vi "Error Enqueue.vi"(6 "Priority?":bool, 8 "error in":errorcluster, 11 "Error Message in":refnum<class "Error.lvclass">) -> (0 "error out":errorcluster, 3 "Error Message out":refnum<class "Error.lvclass">)   [LabVIEW 2017, in "TSC Error.lvlib"]
doc: "Send an error message.\n\nInputs:\n-Error Message in [obj] - the dynamic dispatch input class that will be queued to the Error Loop\n-error in\n\nOutputs:\n-Error Message out [obj] - the dynamic dispatch class that was queued to the Error Loop\n-error out\n________________________________________________________________________________\n<b>Code Developed By:</b>\nDaniel Coons\nTechnology Service Corporation\n1983 S Liberty Drive\nBloomington, IN 47403\nPhone: 812 558-7100\ndaniel.coons@tsc.com\nwww.tsc.com\n\n<b>Date Created:</b> 11 AUG 2014\n<b>Date Updated:</b>"
uses:
  TSC Error.lvlib
  _Messages/Error/Error.lvclass
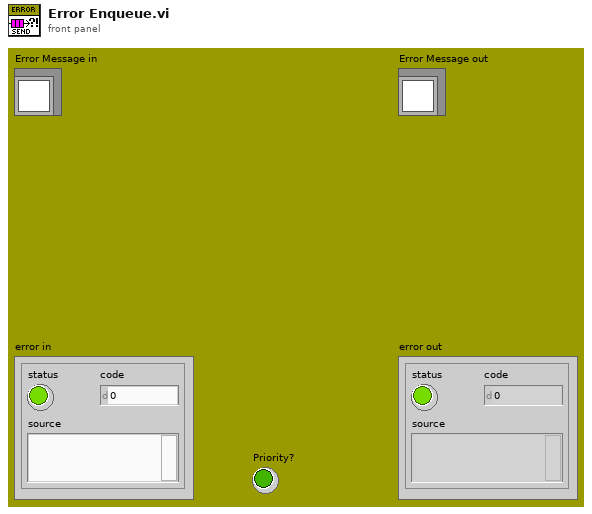
[diagram p1: front panel]
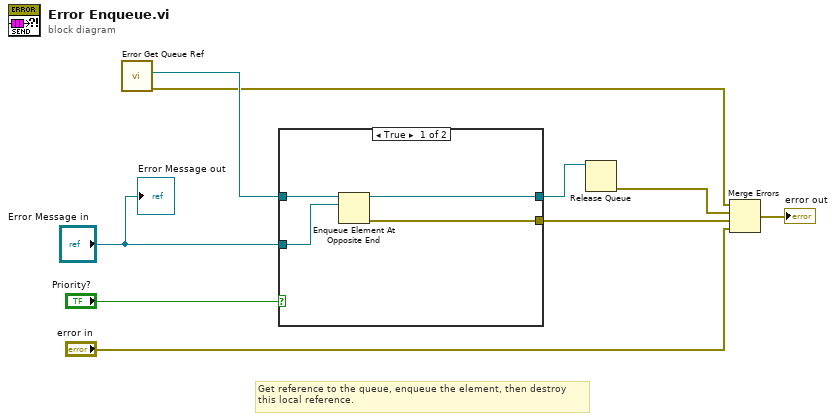
[diagram p0: block diagram]
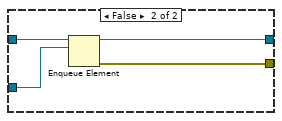
[diagram p2: hidden frame]
diagram:
  # "Get reference to the queue, enqueue the element, then destroy\nthis local reference."
  n1 = call "Error Get Queue Ref.vi"() -> ("error out"=w5:errorcluster, "Error Queue out"=w7:refnum<queue>)  [unwired: 9 in, 1 out]
  n2 = case shown="True" "Priority?" {
    tunnel: "Error Message in" -> [w13 w17]
    tunnel: [w12 w16] -> w4
    tunnel: [w11 w15] -> w8
    tunnel: w7 -> [w10 w14]
    frame True {
      n3 = Enqueue Element At Opposite End(queue=w10, element=w13) -> (queue out=w11:refnum<queue>, error out=w12:errorcluster)  [unwired: 2 in, 1 out]
    }
    frame False {
      n4 = Enqueue Element(queue=w14, element=w17) -> (queue out=w15:refnum<queue>, error out=w16:errorcluster)  [unwired: 2 in, 1 out]
    }
  }
  n5 = Release Queue(queue=w8) -> (error out=w9:errorcluster)  [unwired: 2 in, 2 out]
  n6 = Merge Errors(w5, w9, w4, "error in") -> (→"error out":errorcluster)
  "Error Message out" <- "Error Message in"
